vi "Cluster-Array-FormulaNode.vi"() -> ()   [LabVIEW 2025]
panel:
  out "5th Element":dbl
  out "New Array":dbl[](array[numeric])
  in  "Original Array":dbl[](array[numeric])
  in  "Cluster":cluster{"x":dbl, "Index":dbl, "y":dbl}
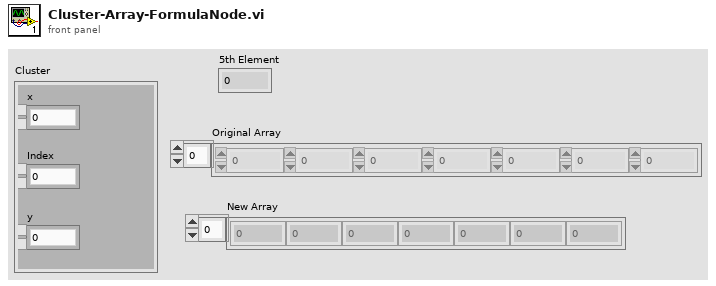
[diagram p1: front panel]
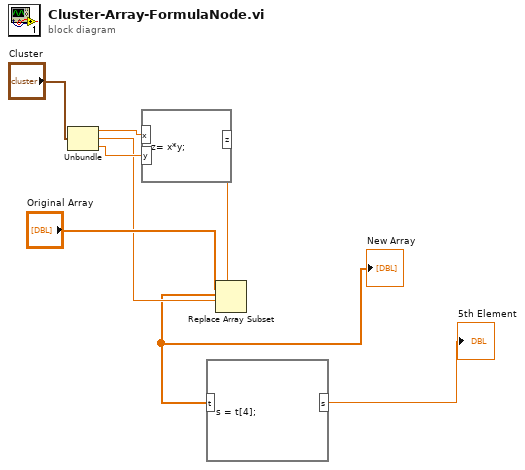
[diagram p0: block diagram]
diagram:
  n1 = Unbundle("Cluster") -> ("x"=w7:dbl, "Index"=w4:dbl, "y"=w6:dbl)
  n2 = formula code="z= x*y;"("x"=w7, "y"=w6) -> ("z"=w3:dbl)
  n3 = Replace Array Subset(array="Original Array", new element=w3, index=w4) -> (w2:dbl[])
  "New Array" <- w2
  n4 = formula code="s = t[4];"("t"=w2) -> ("s"=→"5th Element":dbl)
